vi "Digital Write N Chans.vi"(8 "Error In":errorcluster, 9 "Values":bool[](array[boolean]), 10 "DO Channels":u8[](array[numeric]), 11 "LINX Resource":T1) -> (0 "Error Out":errorcluster, 3 "LINX Resource":T1)   [LabVIEW 2019, in "LMH-LINX.lvlib"]
doc: "Write values to the specified digital output channels."
uses:
  <vilib>/MakerHub/LINX/LMH-LINX.lvlib
  <vilib>/MakerHub/LINX/Private/Type Defs/LINX Ref.ctl
  <vilib>/MakerHub/LINX/Private/Type Defs/Platform.ctl
  <vilib>/MakerHub/LINX/Private/Type Defs/Interface.ctl
  <vilib>/MakerHub/LINX/Private/Device/Type Defs/LINX Device Config.ctl
  <vilib>/MakerHub/LINX/Private/Device/Type Defs/TCP Config.ctl
  <vilib>/MakerHub/LINX/Private/Device/Type Defs/Channels.ctl
  <vilib>/MakerHub/LINX/Private/Type Defs/Peripheral.ctl
  <vilib>/MakerHub/LINX/Private/Utilties/Generate Error.vi
  <vilib>/MakerHub/LINX/Private/Device/Device.lvlib
  <vilib>/MakerHub/LINX/Private/Local IO/Local IO.lvlib
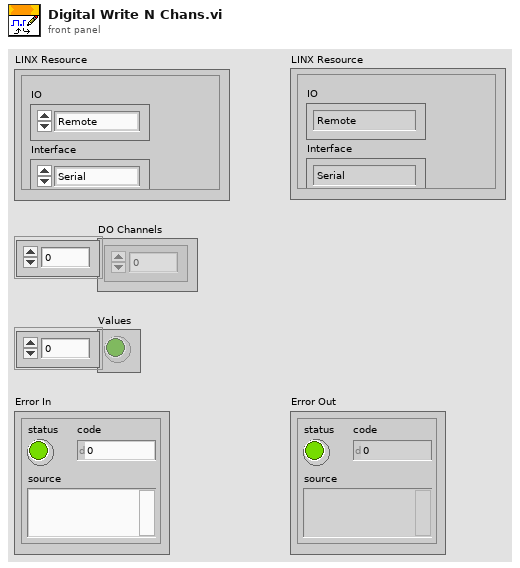
[diagram p1: front panel]
types:
  T1 = typedef "LMH-LINX.lvlib/LINX Ref.ctl" = cluster{"IO":T2, "Interface":T3, "LINX Device Config":T4}
  T2 = typedef "LMH-LINX.lvlib/Platform.ctl" = enum16{"Remote", "Local"}
  T3 = typedef "LMH-LINX.lvlib/Interface.ctl" = enum16{"Serial", "TCP"}
  T4 = typedef "LMH-LINX.lvlib/Device.lvlib/LINX Device Config.ctl" = cluster{"Interface":T3, "COM Port":refnum<visa-resource-name>, "TCP Configuration":T5, "Device Family":u8, "Device ID":u8, "Device Name":string, "TCP Ref":refnum<k5>, "Channels":T6}
  T5 = typedef "LMH-LINX.lvlib/Device.lvlib/TCP Config.ctl" = cluster{"IP Address":string, "Port":u16}
  T6 = typedef "LMH-LINX.lvlib/Channels.ctl" = cluster{"DI":u8[], "DO":u8[], "AI":u8[], "AO":u8[], "PWM":u8[], "QE":u8[], "UART":u8[], "I2C 2":u8[], "SPI":u8[], "CAN":u8[], "Servo":u8[], "AI Ref (V)":dbl, "AI Resolution (Bits)":u8, "AO Ref (V)":dbl, "AO Resolution (Bits)":u8}
  T7 = typedef "LMH-LINX.lvlib/Peripheral.ctl" = enum8{"DI", "DO", "AI", "AO", "PWM", "QE", "UART", "I2C", "SPI", "CAN", "Servo"}
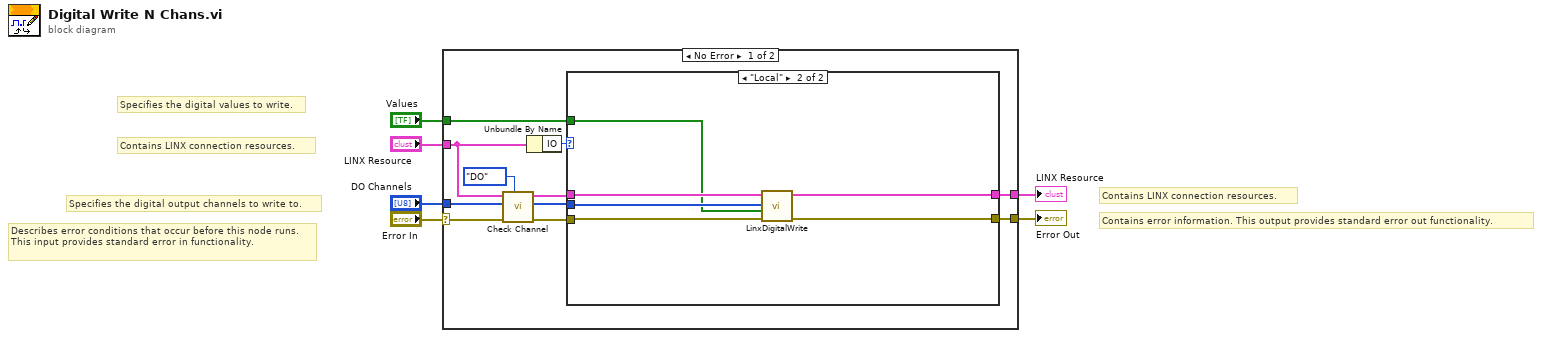
[diagram p0: block diagram]
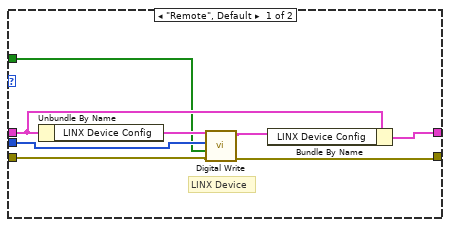
[diagram p2: hidden frame]
diagram:
  # "Specifies the digital output channels to write to."
  # "Specifies the digital values to write."
  # "Contains LINX connection resources."
  # "Contains error information. This output provides standard error out functionality."
  # "Contains LINX connection resources."
  # "Describes error conditions that occur before this node runs. This input provides standard error in functionality."
  n1 = case shown="No Error" "Error In" {
    selector: "Error In" -> [w8 w33]
    tunnel: [w16 w33] -> w6
    tunnel: [w15 w32] -> w5
    tunnel: "LINX Resource" -> [w14 w32]
    tunnel: "DO Channels" -> [w10 _]
    tunnel: "Values" -> [w9 _]
    frame No Error {
      n2 = call <vilib>:"Check Channel.vi"("Peripheral"=Peripheral."DO", "Error In"=w8, "Channels"=w10, "LINX Resource"=w14) -> ("Error Out"=w12:errorcluster, "Channels"=w11:u8[], "LINX Resource"=w13:T1)  [unwired: 5 in]
      n3 = Unbundle By Name(w14) -> ("IO"=w17:T2)
      n4 = case shown="\"Local\"" w17 {
        tunnel: w12 -> [w20 w29]
        tunnel: w13 -> [w25 w31]
        tunnel: [w23 w26] -> w16
        tunnel: [w24 w27] -> w15
        tunnel: w9 -> [w18 w28]
        tunnel: w11 -> [w19 w30]
        frame "Remote", Default {
          # "LINX Device"
          n5 = Unbundle By Name(w25) -> ("LINX Device Config"=w21:T4)
          n6 = call <vilib>:"Digital Write.vi"("Error In"=w20, "Values"=w18, "Channels"=w19, "LINX Device Config"=w21) -> ("Error Out"=w23:errorcluster, "LINX Device Config"=w22:T4)  [unwired: 6 in]
          n7 = Bundle By Name(cluster=w25, "LINX Device Config"=w22) -> (w24:T1)
        }
        frame "Local" {
          n8 = call <vilib>:"LinxDigitalWrite.vi"("Error In"=w29, "Values"=w28, "Channels"=w30, "LINX Resource"=w31) -> ("Error Out"=w26:errorcluster, "LINX Resource"=w27:T1)  [unwired: 6 in]
        }
      }
    }
    frame Error {
    }
  }
  "Error Out" <- w6
  "LINX Resource" <- w5
